vi "Get LabVIEW Version.vi"(0 "Type Of LabVIEW Version Descriptor":u16(ring)=1 items=["Major"=1, "Major.Minor"=2, "Major.Minor.Fix"=3]) -> (4 "LabVIEW Version":string, 6 "LabVIEW Build Version":string)   [LabVIEW 2017, in "CL_G3_VIComponentBuilder.lvlib"]
doc: "Returns the version of LabVIEW in the format \"Major.Minor.Fix\" as specified by the \"Type Of LabVIEW Version Descriptor\"."
uses:
  CL_G3_VIComponentBuilder.lvlib
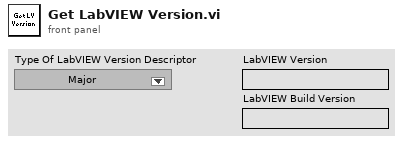
[diagram p1: front panel]
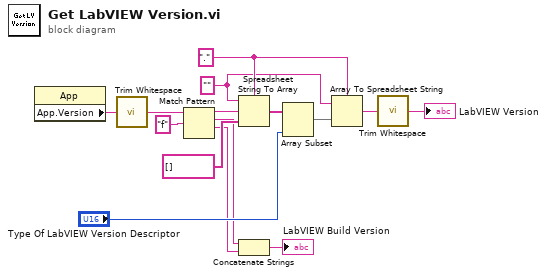
[diagram p0: block diagram]
diagram:
  w10 = "" ("spreadsheet string")
  w11 = "." ("delimiter (Tab)")
  n1 = property class="App"() -> ("App.Version"=w14:string)  [unwired: 2 in, 2 out]
  n2 = call <vilib>:"Trim Whitespace.vi"("string"=w14) -> ("trimmed string"=w2:string)  [unwired: 1 in]
  n3 = Match Pattern(string=w2, regular expression="f") -> (before substring=w1:string, match substring=w6:string, after substring=w5:string)  [unwired: 1 in, 1 out]
  n4 = Spreadsheet String To Array(delimiter (Tab)=w11, format string=w10, spreadsheet string=w1, array type (2D Dbl)=string[] []) -> (array=w13:string[])
  n5 = Concatenate Strings(w6, w5) -> (→"LabVIEW Build Version":string)
  n6 = Array Subset(array=w13, length="Type Of LabVIEW Version Descriptor") -> (w12:string[])  [unwired: 1 in]
  n7 = Array To Spreadsheet String(delimiter (Tab)=w11, array=w12, 3:w10) -> (spreadsheet string=w9:string)
  n8 = call <vilib>:"Trim Whitespace.vi"("string"=w9) -> ("trimmed string"=→"LabVIEW Version":string)  [unwired: 1 in]
